vi "String to Variant.vi"(9 "String":string, 10 "Variable Name":string) -> (2 "variant":variant)   [LabVIEW 2009]
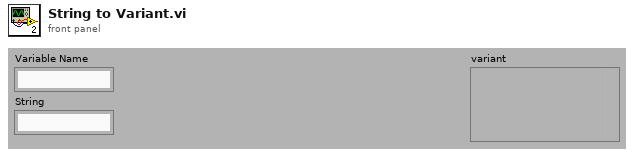
[diagram p1: front panel]
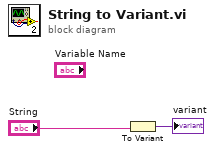
[diagram p0: block diagram]
diagram:
  n1 = To Variant(anything="String") -> (Variant=→"variant":variant)
